vi "CAN自动测试.vi"(10 "选择?":bool) -> ()   [LabVIEW 2010]
uses:
  全局量/试验配置信息.vi
  全局量/自动测试结果.vi
panel:
  in  "同步_2":i32
  in  "同步_1":i32
  out "结束?":bool
  in  "CAN_4_4":u16
  in  "CAN_4_3":u16
  in  "CAN_4_2":u16
  in  "CAN_4_1":u16
  in  "CAN_3_4":u16
  in  "CAN_3_3":u16
  in  "CAN_3_2":u16
  in  "CAN_3_1":u16
  in  "CAN_2_4":u16
  in  "CAN_2_3":u16
  in  "CAN_2_2":u16
  in  "CAN_2_1":u16
  in  "CAN_1_4":u16
  in  "CAN_1_3":u16
  in  "CAN_1_2":u16
  in  "CAN_1_1":u16
  # "CAN1"
  # "CAN2"
  # "CAN3"
  # "CAN4"
  # "测试结论："
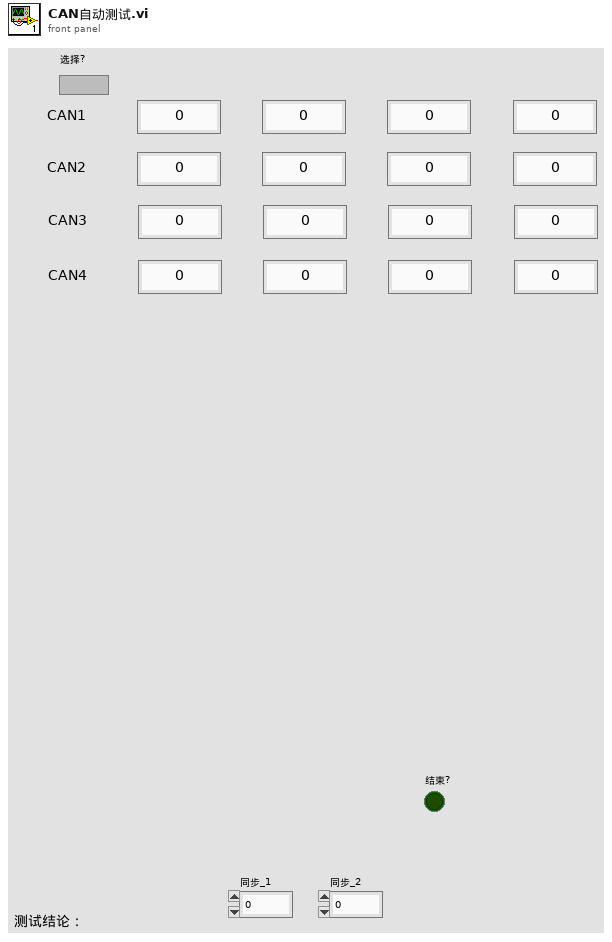
[diagram p1: front panel]
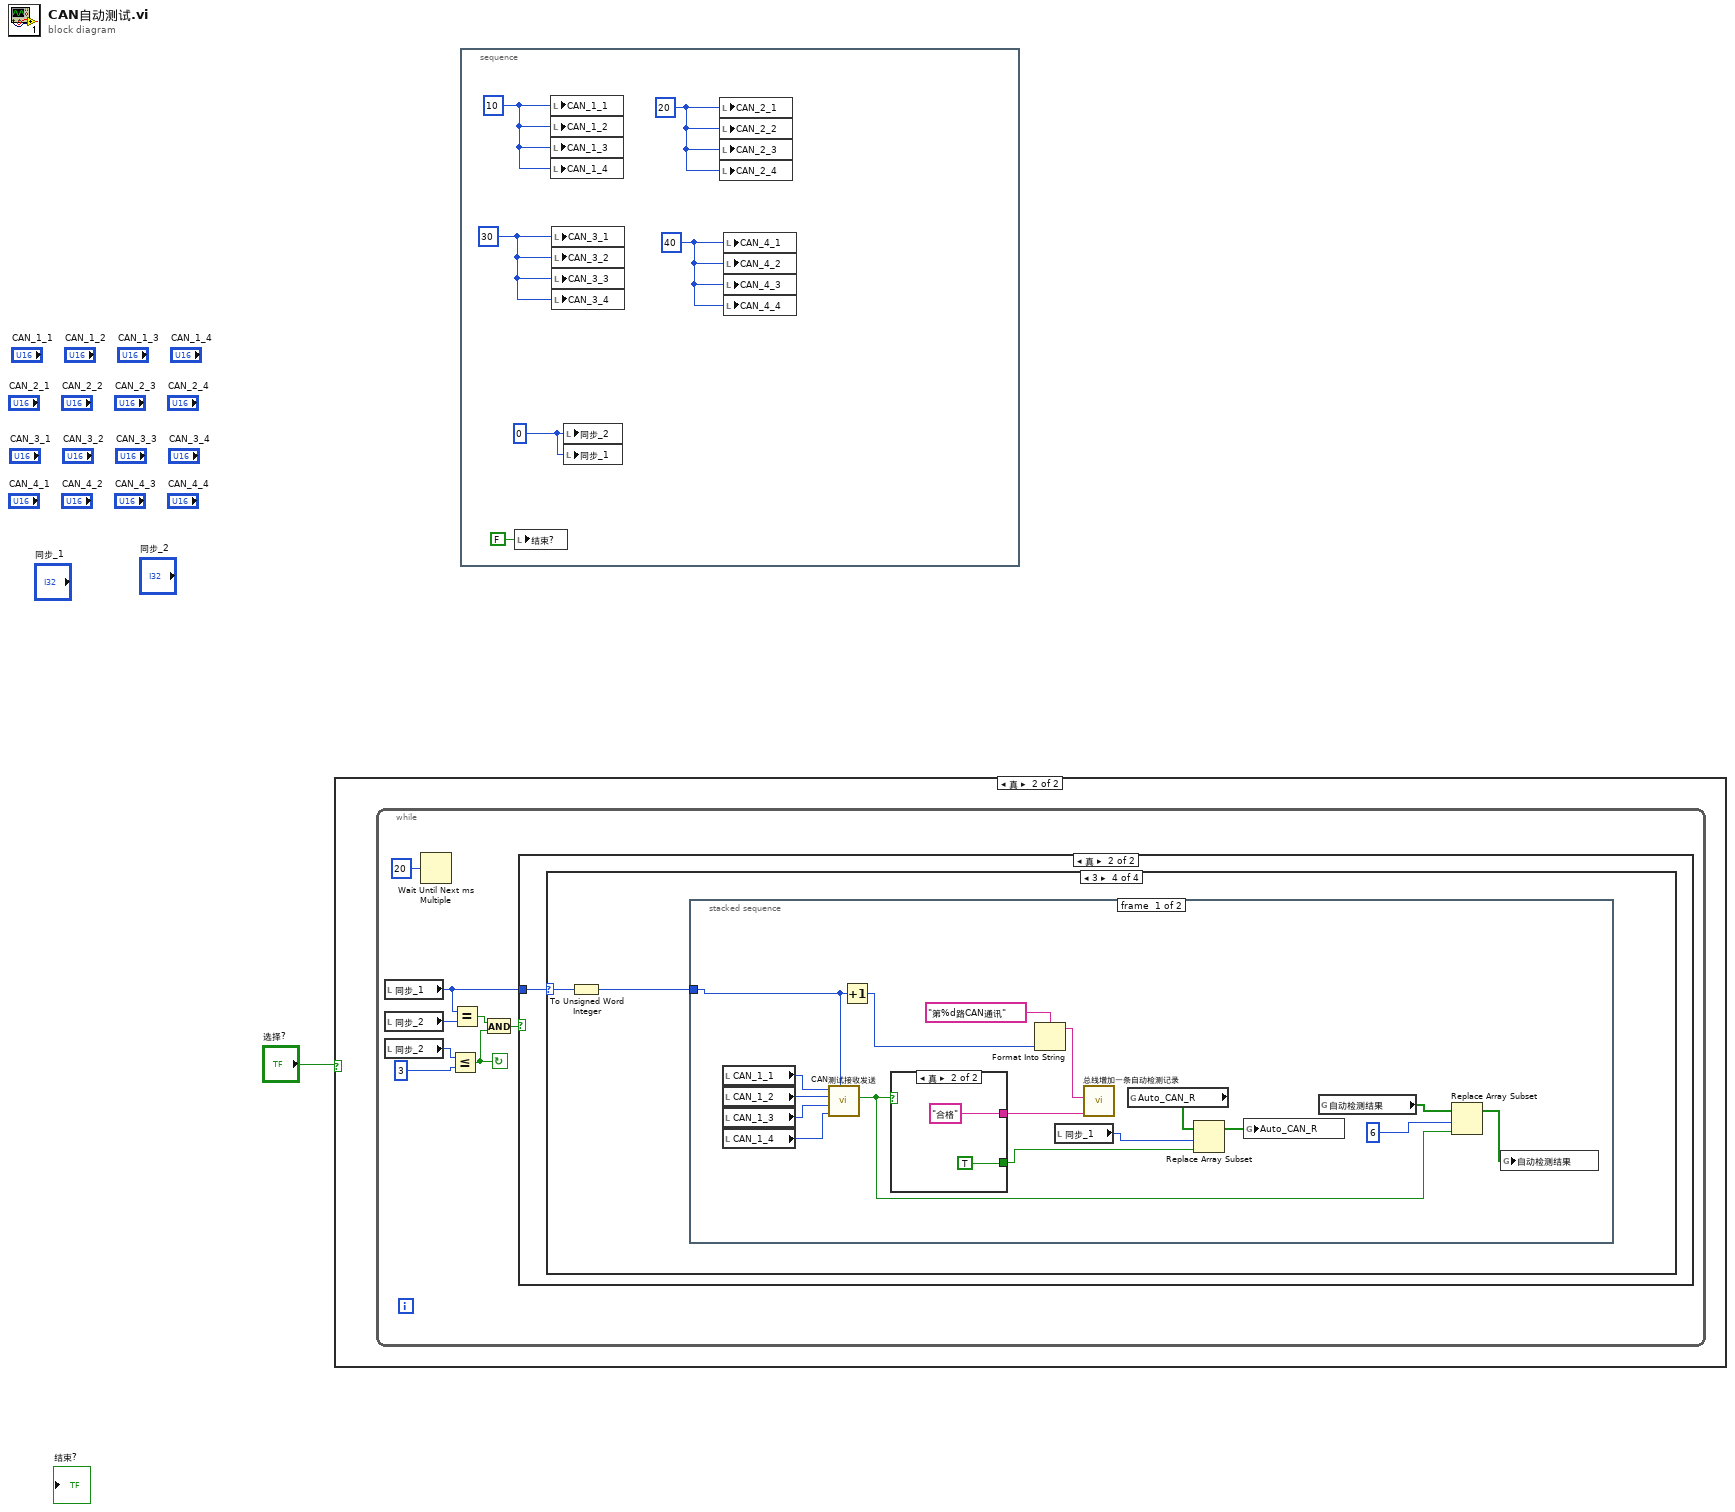
[diagram p0: block diagram]
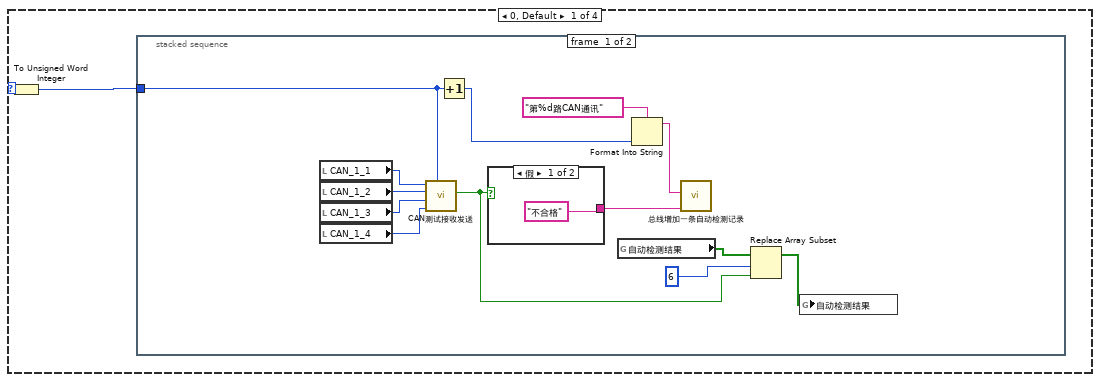
[diagram p4: hidden frame]
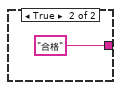
[diagram p5: hidden frame]
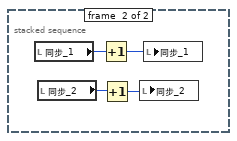
[diagram p6: hidden frame]
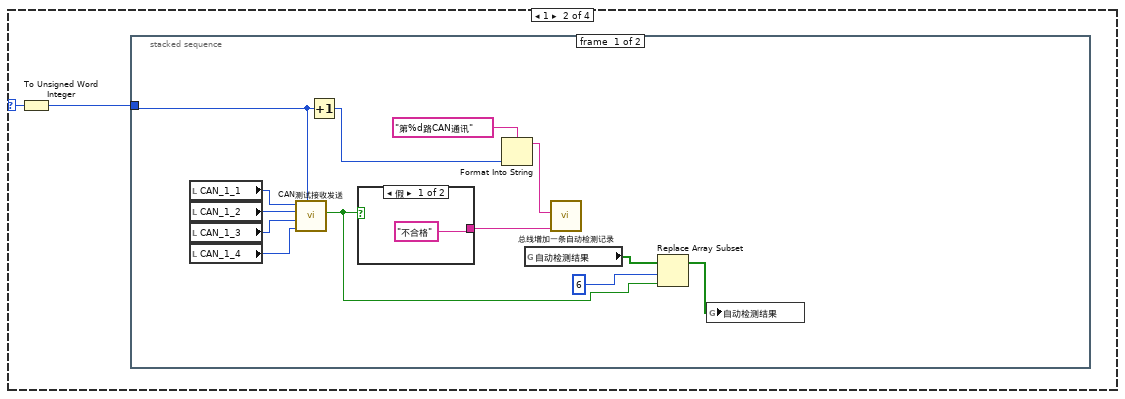
[diagram p7: hidden frame]
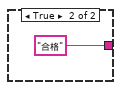
[diagram p8: hidden frame]
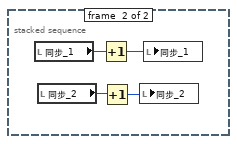
[diagram p9: hidden frame]
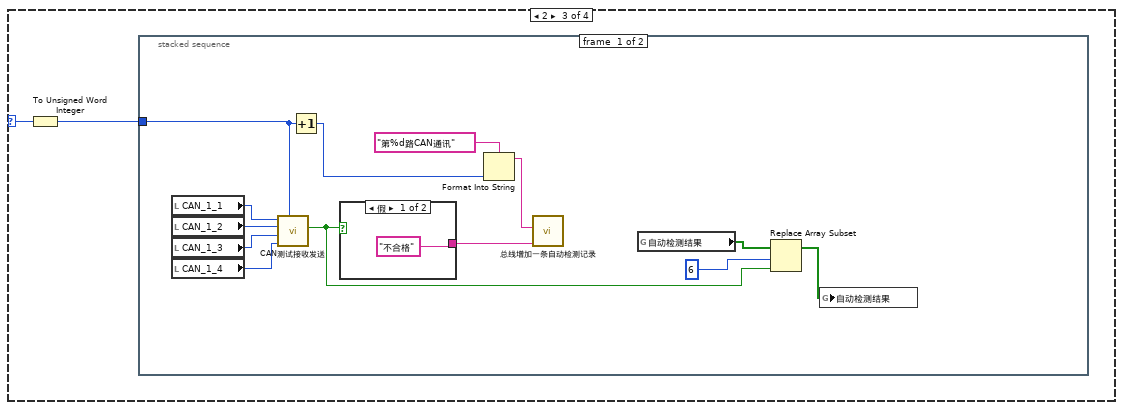
[diagram p10: hidden frame]
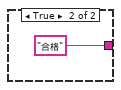
[diagram p11: hidden frame]
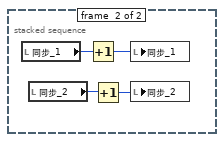
[diagram p12: hidden frame]
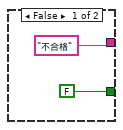
[diagram p13: hidden frame]
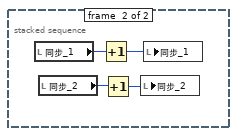
[diagram p14: hidden frame]
diagram:
  n1 = case shown="真" "选择?" {
    frame False {
    }
    frame True {
      n2 = while {
        stop <- w2 continue-if-true
        n3 = local read "同步_1"() -> (w9:i32)
        n4 = local read "同步_2"() -> (w5:i32)
        n5 = local read "同步_2"() -> (w7:i32)
        n6 = Wait Until Next ms Multiple(millisecond multiple=u32 20 ("毫秒倍数")) -> ()  [unwired: 1 out]
        n7 = Less Or Equal?(x=w7, y=3) -> (x <= y?=w2:bool)
        n8 = Equal?(x=w9, y=w5) -> (x = y?=w3:bool)
        n9 = And(x=w3, y=w2) -> (x .and. y?=w4:bool)
        n10 = case shown="真" w4 {
          tunnel: w9 -> [_ w10]
          frame False {
          }
          frame True {
            n11 = case shown="3" w10 {
              selector: w10 -> [w11 w33 w54 w75]
              frame 0, Default {
                n12 = To Unsigned Word Integer(number=w11) -> (unsigned 16bit integer=w12:u16)
                n13 = stacked-sequence {
                  tunnel: w12 -> [w21 _]
                  frame #0 {
                    n14 = local read "CAN_1_1"() -> (w22:u16)
                    n15 = local read "CAN_1_2"() -> (w23:u16)
                    n16 = local read "CAN_1_3"() -> (w24:u16)
                    n17 = local read "CAN_1_4"() -> (w25:u16)
                    n18 = call "CAN测试接收发送.vi"("Order"=w21, "data_4"=w25, "data_3"=w24, "data_2"=w23, "data_1"=w22) -> ("成功？"=w13:bool)  [unwired: 5 in, 1 out]
                    n19 = Increment(x=w21) -> (x+1=w19:u16)
                    n20 = case shown="假" w13 {
                      tunnel: ["不合格" "合格"] -> w17
                      frame False {
                      }
                      frame True {
                      }
                    }
                    n21 = global read "试验配置信息.vi" "自动检测结果"() -> (w16:bool[])
                    n22 = Format Into String(format string="第%d路CAN通讯", w19) -> (resulting string=w18:string)  [unwired: 2 in, 1 out]
                    n23 = call "总线增加一条自动检测记录.vi"("测试结果"=w17, "测试内容"=w18) -> ()  [unwired: 10 in]
                    n24 = Replace Array Subset(array=w16, new element=w13, index=6 ("索引")) -> (w15:bool[])
                    n25 = global write "试验配置信息.vi" "自动检测结果"(w15) -> ()
                  }
                  frame #1 {
                    n26 = local read "同步_1"() -> (w30:i32)
                    n27 = local read "同步_2"() -> (w28:i32)
                    n28 = Increment(x=w30) -> (x+1=w31:i32)
                    n29 = Increment(x=w28) -> (x+1=w29:i32)
                    n30 = local write "同步_2"(w29) -> ()
                    n31 = local write "同步_1"(w31) -> ()
                  }
                }
              }
              frame 1 {
                n32 = To Unsigned Word Integer(number=w33) -> (unsigned 16bit integer=w32:u16)
                n33 = stacked-sequence {
                  tunnel: w32 -> [w38 _]
                  frame #0 {
                    n34 = local read "CAN_1_1"() -> (w43:u16)
                    n35 = local read "CAN_1_2"() -> (w44:u16)
                    n36 = local read "CAN_1_3"() -> (w45:u16)
                    n37 = local read "CAN_1_4"() -> (w46:u16)
                    n38 = call "CAN测试接收发送.vi"("Order"=w38, "data_4"=w46, "data_3"=w45, "data_2"=w44, "data_1"=w43) -> ("成功？"=w34:bool)  [unwired: 5 in, 1 out]
                    n39 = Increment(x=w38) -> (x+1=w41:u16)
                    n40 = case shown="假" w34 {
                      tunnel: ["不合格" "合格"] -> w39
                      frame False {
                      }
                      frame True {
                      }
                    }
                    n41 = Format Into String(format string="第%d路CAN通讯", w41) -> (resulting string=w40:string)  [unwired: 2 in, 1 out]
                    n42 = global read "试验配置信息.vi" "自动检测结果"() -> (w37:bool[])
                    n43 = call "总线增加一条自动检测记录.vi"("测试结果"=w39, "测试内容"=w40) -> ()  [unwired: 10 in]
                    n44 = Replace Array Subset(array=w37, new element=w34, index=6 ("索引")) -> (w36:bool[])
                    n45 = global write "试验配置信息.vi" "自动检测结果"(w36) -> ()
                  }
                  frame #1 {
                    n46 = local read "同步_1"() -> (w51:i32)
                    n47 = local read "同步_2"() -> (w50:i32)
                    n48 = Increment(x=w51) -> (x+1=w52:i32)
                    n49 = Increment(x=w50) -> (x+1=w49:i32)
                    n50 = local write "同步_2"(w49) -> ()
                    n51 = local write "同步_1"(w52) -> ()
                  }
                }
              }
              frame 2 {
                n52 = To Unsigned Word Integer(number=w54) -> (unsigned 16bit integer=w53:u16)
                n53 = stacked-sequence {
                  tunnel: w53 -> [w59 _]
                  frame #0 {
                    n54 = local read "CAN_1_1"() -> (w64:u16)
                    n55 = local read "CAN_1_2"() -> (w65:u16)
                    n56 = local read "CAN_1_3"() -> (w66:u16)
                    n57 = local read "CAN_1_4"() -> (w67:u16)
                    n58 = call "CAN测试接收发送.vi"("Order"=w59, "data_4"=w67, "data_3"=w66, "data_2"=w65, "data_1"=w64) -> ("成功？"=w55:bool)  [unwired: 5 in, 1 out]
                    n59 = Increment(x=w59) -> (x+1=w62:u16)
                    n60 = case shown="假" w55 {
                      tunnel: ["不合格" "合格"] -> w60
                      frame False {
                      }
                      frame True {
                      }
                    }
                    n61 = Format Into String(format string="第%d路CAN通讯", w62) -> (resulting string=w61:string)  [unwired: 2 in, 1 out]
                    n62 = call "总线增加一条自动检测记录.vi"("测试结果"=w60, "测试内容"=w61) -> ()  [unwired: 10 in]
                    n63 = global read "试验配置信息.vi" "自动检测结果"() -> (w58:bool[])
                    n64 = Replace Array Subset(array=w58, new element=w55, index=6 ("索引")) -> (w57:bool[])
                    n65 = global write "试验配置信息.vi" "自动检测结果"(w57) -> ()
                  }
                  frame #1 {
                    n66 = local read "同步_1"() -> (w72:i32)
                    n67 = local read "同步_2"() -> (w70:i32)
                    n68 = Increment(x=w72) -> (x+1=w73:i32)
                    n69 = Increment(x=w70) -> (x+1=w71:i32)
                    n70 = local write "同步_1"(w73) -> ()
                    n71 = local write "同步_2"(w71) -> ()
                  }
                }
              }
              frame 3 {
                n72 = To Unsigned Word Integer(number=w75) -> (unsigned 16bit integer=w74:u16)
                n73 = stacked-sequence {
                  tunnel: w74 -> [w84 _]
                  frame #0 {
                    n74 = local read "CAN_1_1"() -> (w89:u16)
                    n75 = local read "CAN_1_2"() -> (w90:u16)
                    n76 = local read "CAN_1_3"() -> (w91:u16)
                    n77 = local read "CAN_1_4"() -> (w92:u16)
                    n78 = call "CAN测试接收发送.vi"("Order"=w84, "data_4"=w92, "data_3"=w91, "data_2"=w90, "data_1"=w89) -> ("成功？"=w76:bool)  [unwired: 5 in, 1 out]
                    n79 = Increment(x=w84) -> (x+1=w87:u16)
                    n80 = case shown="真" w76 {
                      tunnel: ["不合格" "合格"] -> w85
                      tunnel: [FALSE TRUE] -> w80
                      frame False {
                      }
                      frame True {
                      }
                    }
                    n81 = Format Into String(format string="第%d路CAN通讯", w87) -> (resulting string=w86:string)  [unwired: 2 in, 1 out]
                    n82 = local read "同步_1"() -> (w81:i32)
                    n83 = call "总线增加一条自动检测记录.vi"("测试结果"=w85, "测试内容"=w86) -> ()  [unwired: 10 in]
                    n84 = global read "自动测试结果.vi" "Auto_CAN_R"() -> (w83:bool[])
                    n85 = Replace Array Subset(array=w83, new element=w80, index=w81) -> (w82:bool[])
                    n86 = global write "自动测试结果.vi" "Auto_CAN_R"(w82) -> ()
                    n87 = global read "试验配置信息.vi" "自动检测结果"() -> (w79:bool[])
                    n88 = Replace Array Subset(array=w79, new element=w76, index=6 ("索引")) -> (w78:bool[])
                    n89 = global write "试验配置信息.vi" "自动检测结果"(w78) -> ()
                  }
                  frame #1 {
                    n90 = local read "同步_1"() -> (w100:i32)
                    n91 = local read "同步_2"() -> (w97:i32)
                    n92 = Increment(x=w100) -> (x+1=w99:i32)
                    n93 = Increment(x=w97) -> (x+1=w98:i32)
                    n94 = local write "同步_2"(w98) -> ()
                    n95 = local write "同步_1"(w99) -> ()
                  }
                }
              }
            }
          }
        }
      }
    }
  }
  n96 = stacked-sequence {
    frame #0 {
      w101 = u16 30 ("CAN_R_3_1")
      w102 = u16 40 ("CAN_R_4_1")
      w103 = u16 20 ("CAN_R_2_1")
      w104 = u16 10 ("CAN_R_1_1")
      w105 = 0 ("同步_2")
      n97 = local write "结束?"(FALSE ("结束?")) -> ()
      n98 = local write "CAN_1_1"(w104) -> ()
      n99 = local write "CAN_1_2"(w104) -> ()
      n100 = local write "CAN_1_3"(w104) -> ()
      n101 = local write "CAN_1_4"(w104) -> ()
      n102 = local write "CAN_3_1"(w101) -> ()
      n103 = local write "CAN_3_2"(w101) -> ()
      n104 = local write "CAN_3_3"(w101) -> ()
      n105 = local write "CAN_3_4"(w101) -> ()
      n106 = local write "同步_2"(w105) -> ()
      n107 = local write "同步_1"(w105) -> ()
      n108 = local write "CAN_2_1"(w103) -> ()
      n109 = local write "CAN_2_2"(w103) -> ()
      n110 = local write "CAN_2_3"(w103) -> ()
      n111 = local write "CAN_2_4"(w103) -> ()
      n112 = local write "CAN_4_1"(w102) -> ()
      n113 = local write "CAN_4_2"(w102) -> ()
      n114 = local write "CAN_4_3"(w102) -> ()
      n115 = local write "CAN_4_4"(w102) -> ()
    }
  }
